vi "DummyDestructor.vi"(0 "reference in":refnum<class "G#RealTimeTemplate.lvclass">, 5 "error in (no error)":errorcluster) -> (14 "reference out":refnum<class "G#RealTimeTemplate.lvclass">, 19 "error out":errorcluster)   [LabVIEW 2020, in "G#RealTimeTemplate.lvclass"]
doc: "Destroctor"
uses:
  <vilib>/addons/_AddQ/G#Templates/G#RealTimeTemplate/G#RealTimeTemplate.lvclass
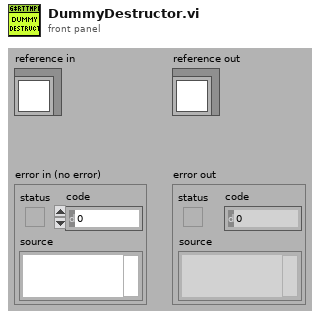
[diagram p1: front panel]
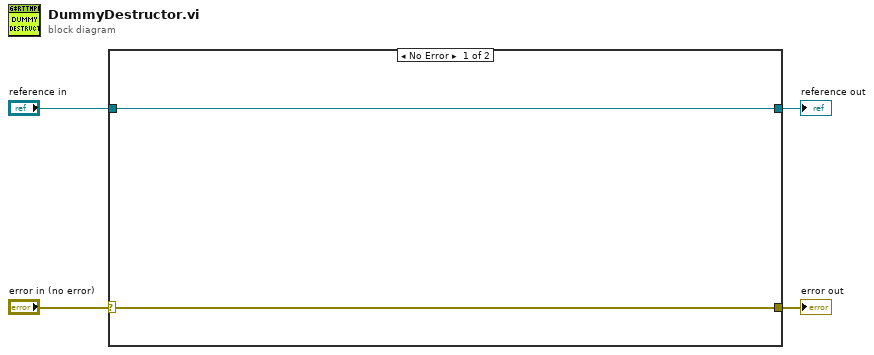
[diagram p0: block diagram]
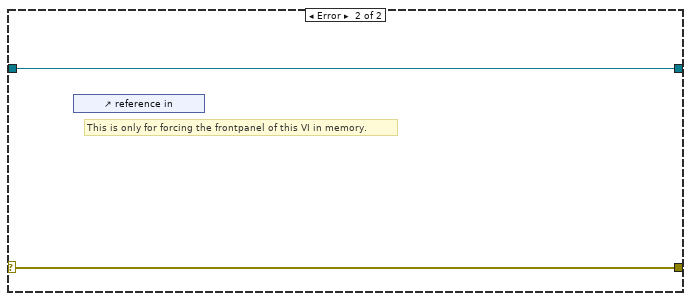
[diagram p2: hidden frame]
diagram:
  n1 = case shown="No Error" "error in (no error)" {
    selector: "error in (no error)" -> [w5 w8]
    tunnel: [w5 w8] -> w3
    tunnel: [w6 w7] -> w1
    tunnel: "reference in" -> [w6 w7]
    frame No Error {
    }
    frame Error {
      # "This is only for forcing the frontpanel of this VI in memory."
      n2 = control-ref of="reference in"() -> ()  [unwired: 1 out]
    }
  }
  "error out" <- w3
  "reference out" <- w1
